vi "add vis to folder.vi"(8 "error in":errorcluster, 10 "startup":path[](array[path]), 11 "ProjectItem in":refnum<vi>) -> (0 "error out":errorcluster, 3 "ids":string[](array[string]))   [LabVIEW 2013]
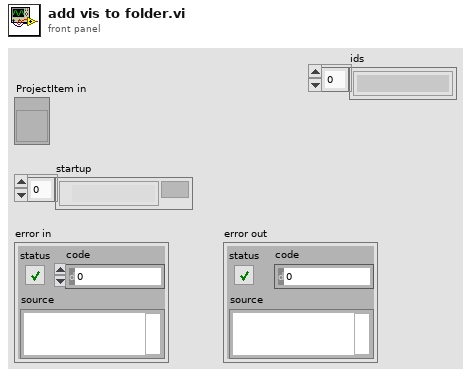
[diagram p1: front panel]
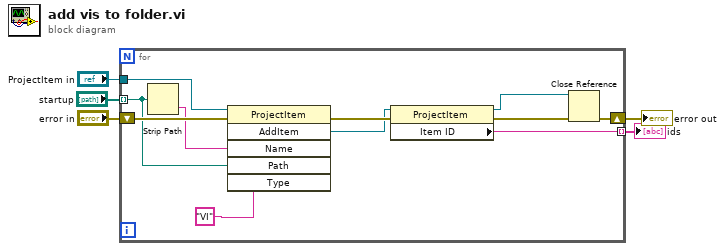
[diagram p0: block diagram]
diagram:
  n1 = for {
    tunnel: "ProjectItem in" -> [w14]
    shift-right: [w15] -> w5
    shift-left: "error in" -> [w16]
    tunnel: "startup" -> [w11] mode=indexing
    tunnel: [w6] -> w1 mode=indexing
    n2 = Strip Path(path=w11) -> (name=w12:string)  [unwired: 1 out]
    n3 = invoke class="ProjectItem" method="AddItem"(reference=w14, error in=w16, "Name"=w12, "Path"=w11, "Type"="VI") -> (error out=w10:errorcluster, "AddItem"=w9:refnum<vi>)  [unwired: 1 in, 4 out]
    n4 = property class="ProjectItem"(reference=w9, error in=w10) -> (reference out=w7:refnum<vi>, error out=w8:errorcluster, "Item ID"=w6:string)
    n5 = Close Reference(reference=w7, error in (no error)=w8) -> (error out=w15:errorcluster)
  }
  "error out" <- w5
  "ids" <- w1
